vi "Aggregate.vi"(10 "matches":bool[](array[boolean]), 11 "filter":refnum<class "Filter.lvclass">) -> (2 "match?":bool, 3 "dup filter":refnum<class "Filter.lvclass">)   [LabVIEW 2024, in "Logging.lvlib" / "Filter.lvclass"]
uses:
  Filter.lvclass
  Filter.lvclass/Filter.ctl
panel:
  # "Connector Pane"
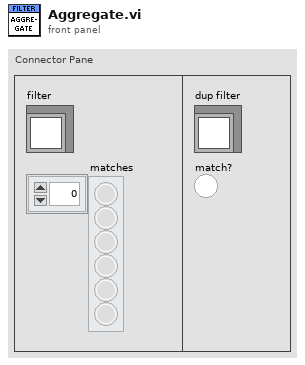
[diagram p1: front panel]
types:
  T1 = typedef "Logging.lvlib/Aggregation Method.ctl" = enum16{"Any", "Only", "All", "None"}
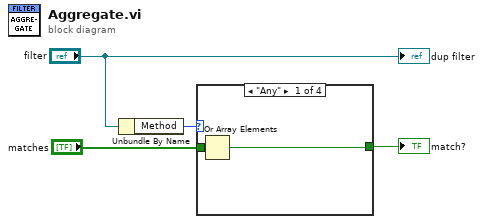
[diagram p0: block diagram]
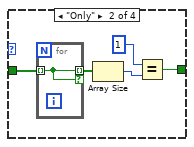
[diagram p2: hidden frame]
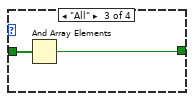
[diagram p3: hidden frame]
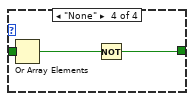
[diagram p4: hidden frame]
diagram:
  n1 = Unbundle By Name("filter") -> ("Method"=w1:T1)
  n2 = case shown="\"Any\"" w1 {
    tunnel: "matches" -> [w6 w11 w14 w17]
    tunnel: [w5 w7 w13 w15] -> w3
    frame "Any" {
      n3 = Or Array Elements(Boolean array=w6) -> (logical OR=w5:bool)
    }
    frame "Only" {
      n4 = for {
        tunnel: w11 -> [w12] mode=indexing
        tunnel: [w12] -> w10 mode=indexing if=w12
      }
      n5 = Array Size(array=w10) -> (size(s)=w9:i32)
      n6 = Equal?(x=1, y=w9) -> (x = y?=w7:bool)
    }
    frame "All" {
      n7 = And Array Elements(Boolean array=w14) -> (logical AND=w13:bool)
    }
    frame "None" {
      n8 = Or Array Elements(Boolean array=w17) -> (logical OR=w16:bool)
      n9 = Not(x=w16) -> (.not. x?=w15:bool)
    }
  }
  "match?" <- w3
  "dup filter" <- "filter"
